vi "Set Plot limits.vi"(1 "Min":dbl, 2 "Max":dbl) -> (0 "resulting string":string)   [LabVIEW 2022 SP3]
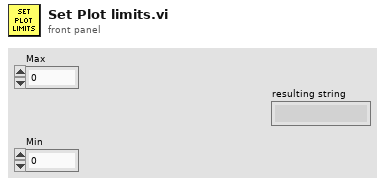
[diagram p1: front panel]
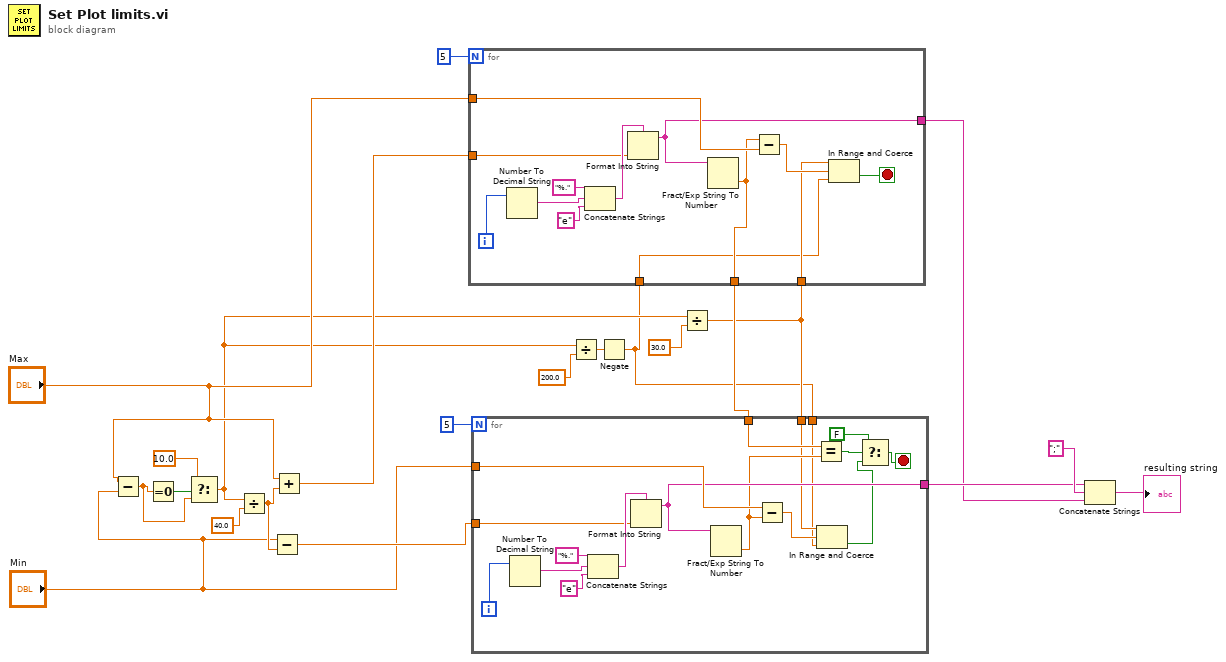
[diagram p0: block diagram]
diagram:
  n1 = Subtract(x="Max", y="Min") -> (x-y=w18:dbl)
  n2 = Equal To 0?(x=w18) -> (x = 0?=w19:bool)
  n3 = Select(t=10.0, s=w19, f=w18) -> (s? t:f=w5:dbl)
  n4 = Divide(x=w5, y=40.0) -> (x/y=w20:dbl)
  n5 = Subtract(x="Min", y=w20) -> (x-y=w13:dbl)
  n6 = Add(x="Max", y=w20) -> (x+y=w15:dbl)
  n7 = Divide(x=w5, y=200.0) -> (x/y=w3:dbl)
  n8 = Negate(x=w3) -> (-x=w1:dbl)
  n9 = Divide(x=w5, y=30.0) -> (x/y=w2:dbl)
  n10 = for {
    N: 5 -> [_]
    tunnel: w15 -> [w30]
    tunnel: "Max" -> [w29]
    tunnel: [w28] -> w8
    tunnel: [w27] -> w7
    tunnel: w2 -> [w25]
    tunnel: w1 -> [w24]
    i -> [w32]
    stop <- w23 stop-if-true
    n11 = Number To Decimal String(number=w32) -> (decimal integer string=w35:string)  [unwired: 1 in]
    n12 = Concatenate Strings("%." ("format string"), w35, "e" ("format string")) -> (w31:string)
    n13 = Format Into String(format string=w31, w30) -> (resulting string=w28:string)  [unwired: 2 in, 1 out]
    n14 = Fract/Exp String To Number(string=w28) -> (number=w27:dbl)  [unwired: 3 in, 1 out]
    n15 = Subtract(x=w27, y=w29) -> (x-y=w26:dbl)
    n16 = In Range and Coerce(upper limit=w25, x=w26, lower limit=w24) -> (In Range?=w23:bool)  [unwired: 1 out]
  }
  n17 = for {
    N: 5 -> [_]
    tunnel: w13 -> [w47]
    tunnel: "Min" -> [w46]
    tunnel: [w44] -> w9
    tunnel: w7 -> [w45]
    tunnel: w2 -> [w37]
    tunnel: w1 -> [w36]
    i -> [w49]
    stop <- w41 stop-if-true
    n18 = Number To Decimal String(number=w49) -> (decimal integer string=w52:string)  [unwired: 1 in]
    n19 = Concatenate Strings("%." ("format string"), w52, "e" ("format string")) -> (w48:string)
    n20 = Format Into String(format string=w48, w47) -> (resulting string=w44:string)  [unwired: 2 in, 1 out]
    n21 = Fract/Exp String To Number(string=w44) -> (number=w40:dbl)  [unwired: 3 in, 1 out]
    n22 = Subtract(x=w46, y=w40) -> (x-y=w39:dbl)
    n23 = Equal?(x=w45, y=w40) -> (x = y?=w43:bool)
    n24 = In Range and Coerce(upper limit=w37, x=w39, lower limit=w36) -> (In Range?=w38:bool)  [unwired: 1 out]
    n25 = Select(t=FALSE, s=w43, f=w38) -> (s? t:f=w41:bool)
  }
  n26 = Concatenate Strings(w9, ";" ("string"), w8) -> (→"resulting string":string)
